vi "Graph_Peak_testing.vi"(0 "Channel Select":u16(ring) items=["Temperature"=9, "Flow/Min"=6, "Pressure_Bar"=3], 1 "CHL":T1={"chl1 MIN"=110.0, "chl1 MAX"=130.0, "chl1 thrshold"=120.0}, 5 "error in":errorcluster, 6 "CSV file path":path) -> (7 "samples count":i32, 9 "Max or peak value":ext[](array[numeric]), 10 "size(s)":i32, 11 "Min or Valley value":ext[](array[numeric]), 12 "Peak_valley_point":ext[](array[numeric]), 13 "Peak_valley_point_time":timestamp[](array[timestamp]), 14 "Max Valley/Min":dbl, 15 "XY Graph 2":cluster{timestamp[], ext[]}(graph), 17 "Min Valley/Min":dbl, 18 "Peak or Valley Fail":bool, 19 "error out":errorcluster)   [LabVIEW 2017]
uses:
  <vilib>/Utility/miscctls.llb/LVCursorListTypeDef.ctl
  <vilib>/Utility/file.llb/Read Delimited Spreadsheet (string).vi
  <userlib>/_OpenG.lib/array/array.llb/Remove Duplicates from 1D Array (Variant)__ogtk.vi
  <userlib>/_OpenG.lib/array/array.llb/Delete Elements from 1D Array (EXT)__ogtk.vi
panel:
  out "size(s) 5":i32
  out "array w/ subset deleted":ext[](array[numeric]) format="%.2f"
  out "indices of removed elements":i32[](array[numeric])
  out "size(s) 3":i32
  out "Numeric 3":i32
  out "Numeric":i32
  out "Array 13":ext[][](array[numeric])
  out "Array 12":ext[](array[numeric])
  out "deleted portion 2":ext[](array[numeric])
  out "appended array 2":timestamp[][](array[timestamp])
  out "size(s) 2":i32
  out "Array 11":ext[](array[numeric])
  out "Array 8":timestamp[](array[timestamp])
  out "appended array":timestamp[][](array[timestamp])
  out "deleted portion":ext[](array[numeric])
  out "Array 10":ext[](array[numeric])
  out "Array 9":ext[][](array[numeric])
  out "output cluster 3":T2(array[cluster])
  in  "Cursor List 3":T3
  out "Numeric 2":i32
  out "x = y?":bool
  out "x+y 2":i32
  out "STOP THRESHOLD TRIGGER":i32
  out "START THRESHOLD TRIGGER":i32
  out "time stamp":timestamp[](array[timestamp])
  out "number":ext[](array[numeric])
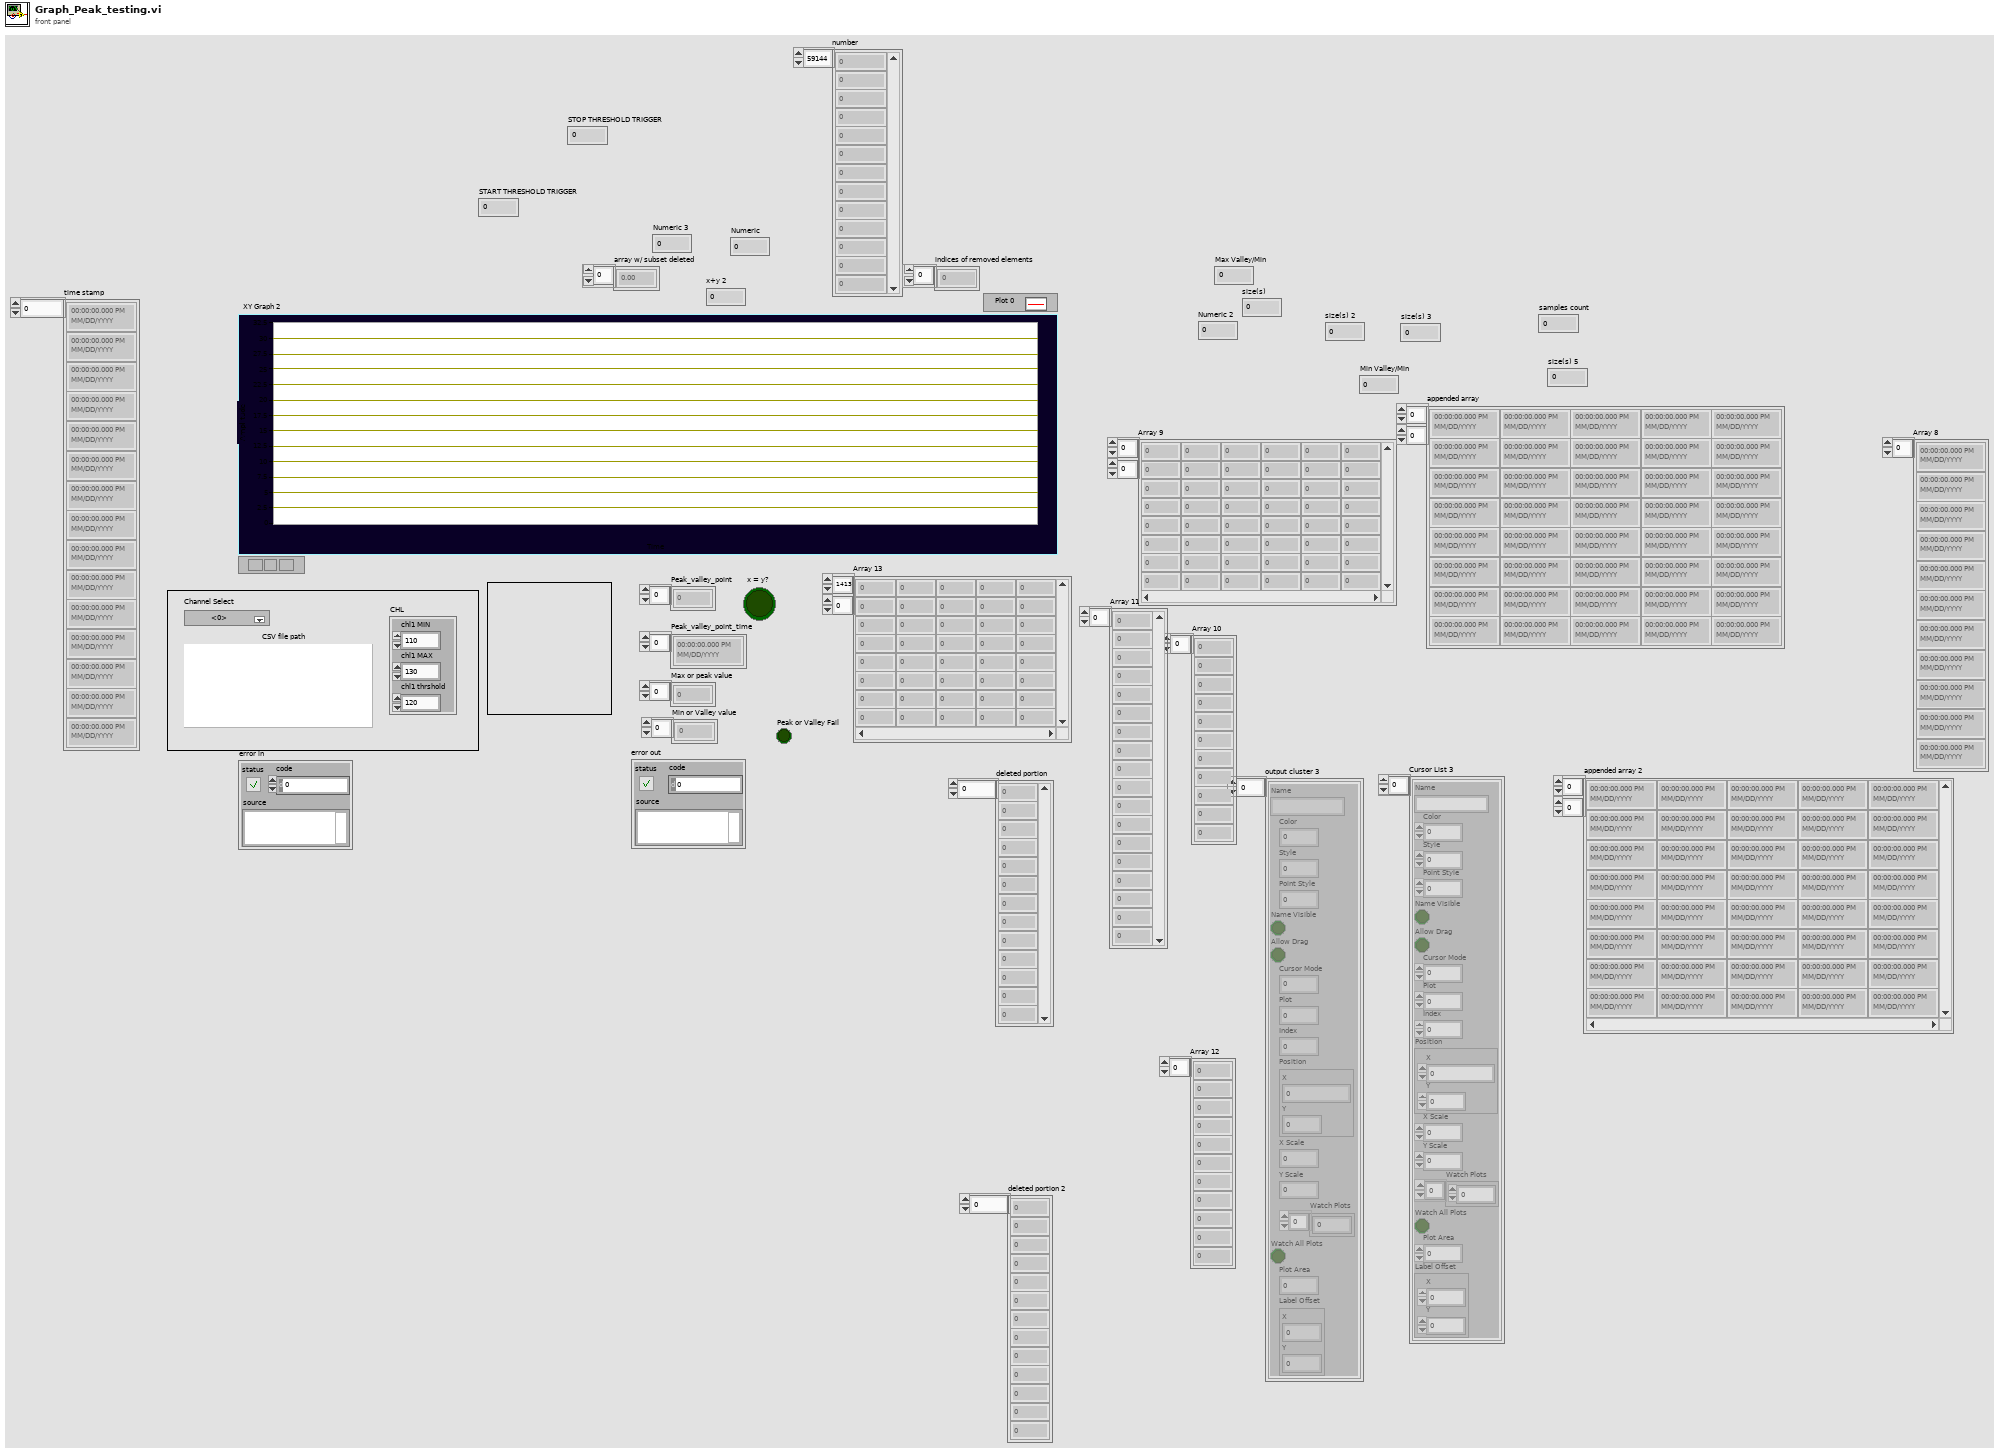
[diagram p1: front panel]
types:
  T1 = cluster{"chl1 MIN":dbl, "chl1 MAX":dbl, "chl1 thrshold":dbl}
  T2 = cluster{"Name":string, "Color":u32, "Style":u8, "Point Style":u8, "Name Visible":bool, "Allow Drag":bool, "Cursor Mode":u32, "Plot":i32, "Index":i32, "Position":cluster{"X":dbl, "Y":dbl}, "X Scale":u32, "Y Scale":u32, "Watch Plots":i32[], "Watch All Plots":bool, "Plot Area":i32, "Label Offset":cluster{"X":dbl, "Y":dbl}}[]
  T3 = typedef "LVCursorListTypeDef.ctl" = cluster{"Name":string, "Color":u32, "Style":u8, "Point Style":u8, "Name Visible":bool, "Allow Drag":bool, "Cursor Mode":u32, "Plot":i32, "Index":i32, "Position":cluster{"X":dbl, "Y":dbl}, "X Scale":u32, "Y Scale":u32, "Watch Plots":i32[], "Watch All Plots":bool, "Plot Area":i32, "Label Offset":cluster{"X":dbl, "Y":dbl}}[]
  T4 = typedef "LVDateTimeRec.ctl" = cluster{"fractional second":dbl, "second":i32, "minute":i32, "hour":i32, "day of month":i32, "month":i32, "year":i32, "day of week":i32, "day of year":i32, "DST":i32}
  T5 = cluster{"Name":string, "Color":u32, "Style":u8, "Point Style":u8, "Name Visible":bool, "Allow Drag":bool, "Cursor Mode":u32, "Plot":i32, "Index":i32, "Position":cluster{"X":dbl, "Y":dbl}, "X Scale":u32, "Y Scale":u32, "Watch Plots":i32[], "Watch All Plots":bool, "Plot Area":i32, "Label Offset":cluster{"X":dbl, "Y":dbl}}
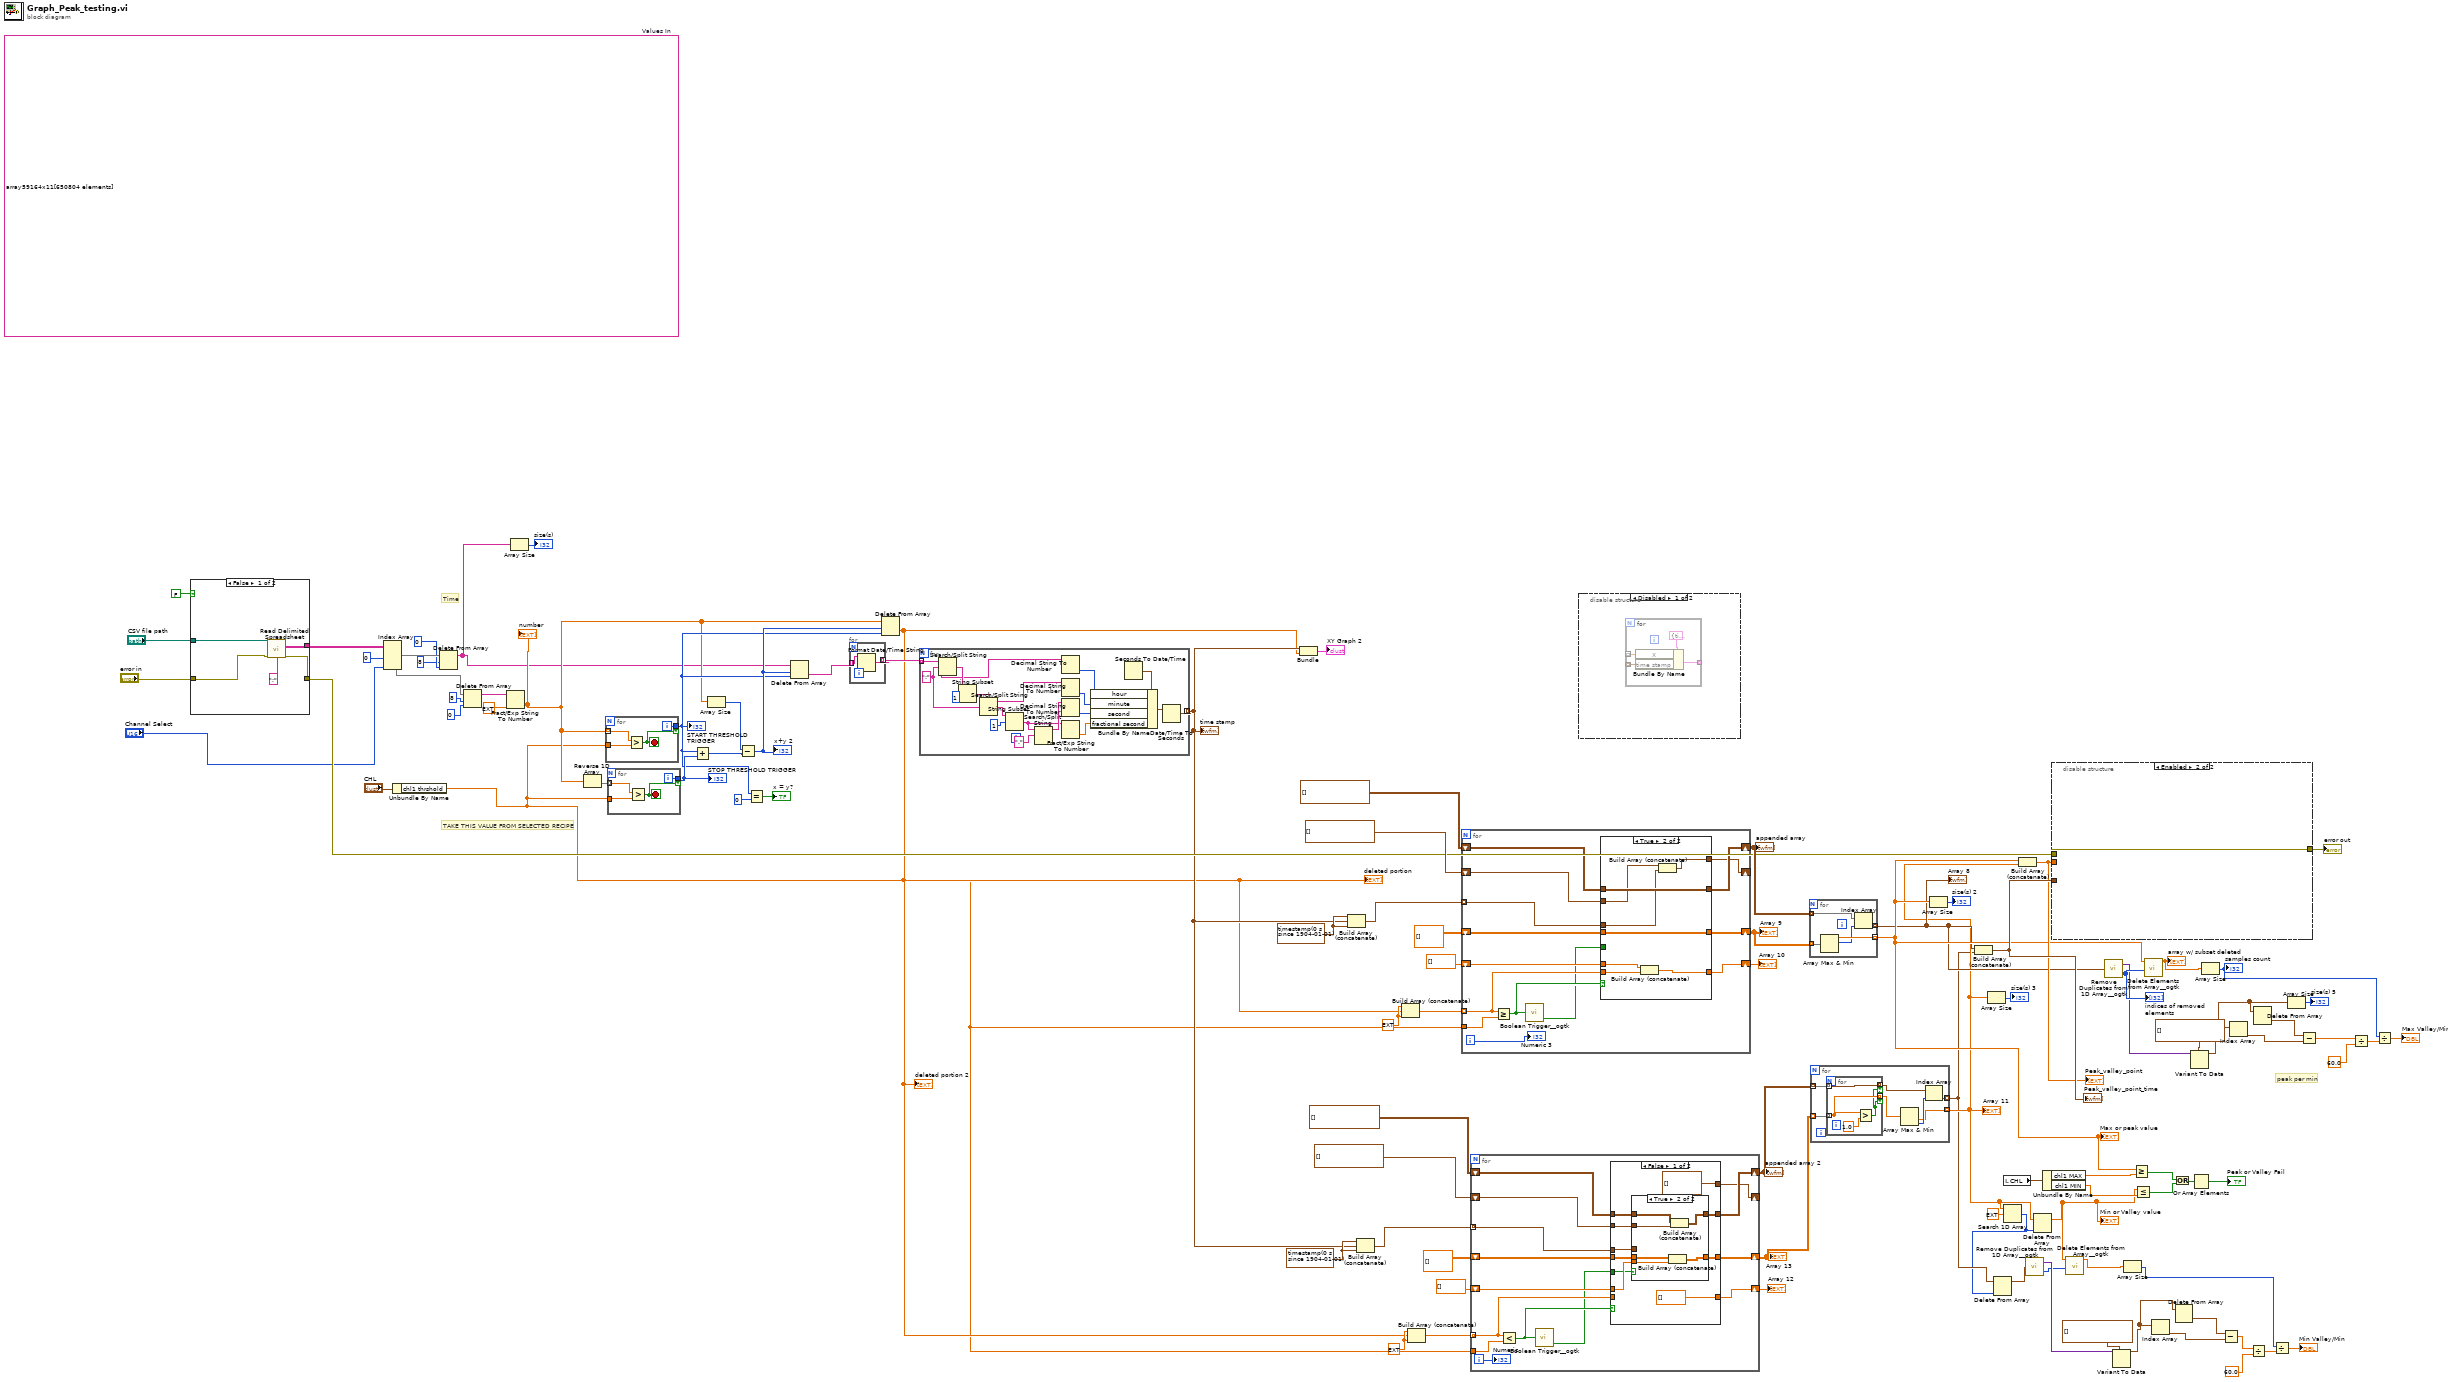
[diagram p0: block diagram]
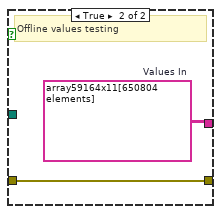
[diagram p3: hidden frame]
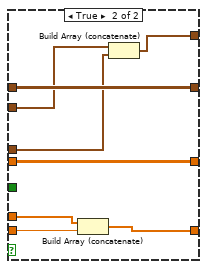
[diagram p5: hidden frame]
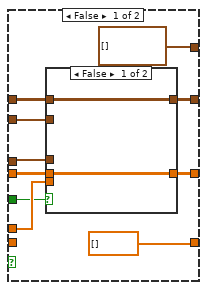
[diagram p6: hidden frame]
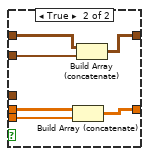
[diagram p7: hidden frame]
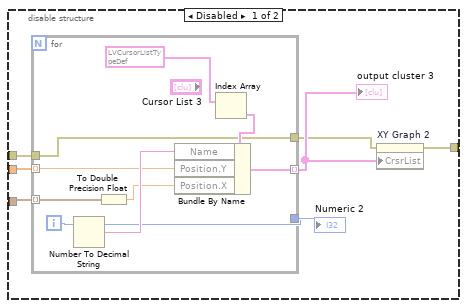
[diagram p8: hidden frame]
diagram:
  (unwired) string[][] array59164x11[650804 elements]  # Values In
  w66 = timestamp(0 s since 1904-01-01) ("time stamp")
  w65 = ext 0.0 ("String")
  w76 = timestamp(0 s since 1904-01-01) ("time stamp")
  w77 = ext 0.0 ("String")
  # "peak per min"
  # "Time"
  # "TAKE THIS VALUE FROM SELECTED RECIPE"
  n1 = case shown="False" FALSE {
    tunnel: [w104 w107] -> w95
    tunnel: "CSV file path" -> [w103 _]
    tunnel: [w102 w106] -> w53
    tunnel: "error in" -> [w101 w106]
    frame False {
      n2 = call-poly <vilib>:"Read Delimited Spreadsheet.vi"("file path (dialog if empty)"=w103, "error in (no error)"=w101, "delimiter (\\t)"=";" ("delimiter (\\t)")) -> ("all rows"=w104:string[][], "error out"=w102:errorcluster)  [unwired: 7 in, 4 out]
    }
    frame True {
      w107 = string[][] array59164x11[650804 elements]  # Values In
      # "Offline values testing"
    }
  }
  n3 = Index Array(array=w95, index (col) #1=0 ("index (row)"), index (col) #2="Channel Select") -> (element #1=w100:string[], element #2=w96:string[])  [unwired: 2 in]
  n4 = Unbundle By Name("CHL") -> ("chl1 thrshold"=w44:dbl)
  n5 = Delete From Array(array=w100, length=8 ("index (row)"), index=0 ("index (row)")) -> (array with subset deleted=w8:string[])  [unwired: 1 out]
  n6 = Delete From Array(array=w96, length=8 ("index (row)"), index=0 ("index (row)")) -> (array with subset deleted=w90:string[])  [unwired: 1 out]
  n7 = Fract/Exp String To Number(string=w90, default (0 dbl)=ext 0.0 ("String")) -> (number=w48:ext[])  [unwired: 2 in, 1 out]
  "number" <- w48
  n8 = Array Size(array=w8) -> (size(s)=→"size(s)":i32)
  n9 = Reverse 1D Array(array=w48) -> (reversed array=w89:ext[])
  n10 = for {
    tunnel: w48 -> [w111] mode=indexing
    tunnel: [w110] -> w84 if=w109
    tunnel: w44 -> [w108]
    i -> [w110]
    stop <- w109 stop-if-true
    n11 = Greater?(x=w111, y=w108) -> (0:w109:bool)
  }
  "START THRESHOLD TRIGGER" <- w84
  n12 = for {
    tunnel: w89 -> [w115] mode=indexing
    tunnel: [w114] -> w88 if=w113
    tunnel: w44 -> [w112]
    i -> [w114]
    stop <- w113 stop-if-true
    n13 = Greater?(x=w115, y=w112) -> (0:w113:bool)
  }
  "STOP THRESHOLD TRIGGER" <- w88
  n14 = Add(x=w84, y=w88) -> (x+y=w86:i32)
  n15 = Array Size(array=w48) -> (size(s)=w87:i32)
  n16 = Subtract(x=w87, y=w86) -> (x-y=w85:i32)
  "x+y 2" <- w85
  n17 = Equal?(x=w84, y=0) -> (x = y?=→"x = y?":bool)
  n18 = Delete From Array(array=w8, length=w85, index=w84) -> (deleted portion=w46:string[])  [unwired: 1 out]
  n19 = for {
    tunnel: w46 -> [w117] mode=indexing
    tunnel: [w116] -> w92 mode=indexing
    n20 = Format Date/Time String(time format string (%c)=w117) -> (date/time string=w116:string)  [unwired: 2 in]
  }
  n21 = Delete From Array(array=w48, length=w85, index=w84) -> (deleted portion=w47:ext[])  [unwired: 1 out]
  "deleted portion" <- w47
  "deleted portion 2" <- w47
  n22 = for {
    tunnel: w92 -> [w126] mode=indexing
    tunnel: [w134] -> w50 mode=indexing
    w133 = ":" ("format string")
    n23 = Search/Split String(string=w126, search string/char (-)=w133) -> (substring before match=w122:string, match + rest of string=w131:string)  [unwired: 1 in, 1 out]
    n24 = String Subset(string=w131, offset (0)=1) -> (substring=w130:string)  [unwired: 1 in]
    n25 = Search/Split String(string=w130, search string/char (-)=w133) -> (substring before match=w121:string, match + rest of string=w128:string)  [unwired: 1 in, 1 out]
    n26 = String Subset(string=w128, offset (0)=1) -> (substring=w120:string)  [unwired: 1 in]
    n27 = Search/Split String(string=w120, search string/char (-)="." ("format string")) -> (substring before match=w125:string)  [unwired: 1 in, 2 out]
    n28 = Decimal String To Number(string=w122) -> (number=w123:i32)  [unwired: 2 in, 1 out]
    n29 = Decimal String To Number(string=w121) -> (number=w124:i32)  [unwired: 2 in, 1 out]
    n30 = Decimal String To Number(string=w125) -> (number=w118:i32)  [unwired: 2 in, 1 out]
    n31 = Fract/Exp String To Number(string=w120) -> (number=w119:dbl)  [unwired: 3 in, 1 out]
    n32 = Seconds To Date/Time() -> (date time rec=w135:T4)  [unwired: 2 in]
    n33 = Bundle By Name(cluster=w135, "hour"=w123, "minute"=w124, "second"=w118, "fractional second"=w119) -> (w136:T4)
    n34 = Date/Time To Seconds(2:w136) -> (0:w134:timestamp)  [unwired: 1 in]
  }
  "time stamp" <- w50
  n35 = Bundle(w50, w47) -> (→"XY Graph 2":cluster{timestamp[], ext[]})  [unwired: 1 in]
  n36 = Build Array (concatenate)(w76, w50, w76) -> (w73:timestamp[])
  n37 = Build Array (concatenate)(w66, w50, w66) -> (w69:timestamp[])
  n38 = Build Array (concatenate)(w77, w47, w77) -> (w78:ext[])
  n39 = Build Array (concatenate)(w65, w47, w65) -> (w64:ext[])
  n40 = for {
    tunnel: w78 -> [w148] mode=indexing
    tunnel: w44 -> [w150]
    shift-right: [w147] -> w79
    shift-left: ext[] [] -> [w146]
    shift-right: [w144] -> w72
    shift-left: ext[][] [] -> [w145]
    tunnel: w73 -> [w142] mode=indexing
    shift-right: [w141] -> w71
    shift-left: timestamp[][] [] ("appended array") -> [w140]
    shift-right: [w138] -> _
    shift-left: timestamp[] [] ("appended array") -> [w139]
    i -> [w137]
    n41 = Greater Or Equal?(x=w148, y=w150) -> (x >= y?=w149:bool)
    n42 = call <userlib>:"Boolean Trigger__ogtk.vi"("Boolean Input"=w149) -> ("Falling Edge"=w143:bool)  [unwired: 1 in, 1 out]
    n43 = case shown="True" w149 {
      tunnel: w148 -> [_ w176]
      tunnel: [ext[] [] w175] -> w147
      tunnel: w146 -> [w157 w173]
      tunnel: w145 -> [w158 w174]
      tunnel: [w159 w174] -> w144
      tunnel: w143 -> [w156 _]
      tunnel: w142 -> [w155 w169]
      tunnel: [w154 w172] -> w141
      tunnel: w140 -> [w153 w172]
      tunnel: w139 -> [w152 w170]
      tunnel: [timestamp[] [] ("appended array") w171] -> w138
      frame False {
        n44 = case shown="False" w156 {
          tunnel: [w162 w168] -> w159
          tunnel: w158 -> [w162 w167]
          tunnel: w157 -> [_ w166]
          tunnel: w155 -> [_ _]
          tunnel: [w161 w165] -> w154
          tunnel: w153 -> [w161 w164]
          tunnel: w152 -> [_ w163]
          frame False {
          }
          frame True {
            n45 = Build Array (concatenate)(w167, w166) -> (w168:ext[][])
            n46 = Build Array (concatenate)(w164, w163) -> (w165:timestamp[][])
          }
        }
      }
      frame True {
        n47 = Build Array (concatenate)(w173, w176) -> (w175:ext[])
        n48 = Build Array (concatenate)(w170, w169) -> (w171:timestamp[])
      }
    }
    "Numeric 3" <- w137
  }
  "Array 9" <- w72
  "Array 10" <- w79
  "appended array" <- w71
  n49 = for {
    tunnel: w64 -> [w188] mode=indexing
    tunnel: w44 -> [w190]
    shift-right: [w187] -> w63
    shift-left: ext[] [] -> [w186]
    shift-right: [w184] -> w58
    shift-left: ext[][] [] -> [w185]
    tunnel: w69 -> [w182] mode=indexing
    shift-right: [w181] -> w57
    shift-left: timestamp[][] [] ("appended array") -> [w180]
    shift-right: [w178] -> _
    shift-left: timestamp[] [] ("appended array") -> [w179]
    i -> [w177]
    n50 = Less?(x=w188, y=w190) -> (x < y?=w189:bool)
    n51 = call <userlib>:"Boolean Trigger__ogtk.vi"("Boolean Input"=w189) -> ("Falling Edge"=w183:bool)  [unwired: 1 in, 1 out]
    n52 = case shown="False" w189 {
      tunnel: w188 -> [_ w216]
      tunnel: [ext[] [] w215] -> w187
      tunnel: w186 -> [w197 w213]
      tunnel: w185 -> [w198 w214]
      tunnel: [w199 w214] -> w184
      tunnel: w183 -> [w196 _]
      tunnel: w182 -> [w195 w209]
      tunnel: [w194 w212] -> w181
      tunnel: w180 -> [w193 w212]
      tunnel: w179 -> [w192 w210]
      tunnel: [timestamp[] [] ("appended array") w211] -> w178
      frame False {
        n53 = case shown="True" w196 {
          tunnel: [w202 w208] -> w199
          tunnel: w198 -> [w202 w207]
          tunnel: w197 -> [_ w206]
          tunnel: w195 -> [_ _]
          tunnel: [w201 w205] -> w194
          tunnel: w193 -> [w201 w204]
          tunnel: w192 -> [_ w203]
          frame False {
          }
          frame True {
            n54 = Build Array (concatenate)(w207, w206) -> (w208:ext[][])
            n55 = Build Array (concatenate)(w204, w203) -> (w205:timestamp[][])
          }
        }
      }
      frame True {
        n56 = Build Array (concatenate)(w213, w216) -> (w215:ext[])
        n57 = Build Array (concatenate)(w210, w209) -> (w211:timestamp[])
      }
    }
    "Numeric" <- w177
  }
  "Array 13" <- w58
  "Array 12" <- w63
  "appended array 2" <- w57
  n58 = disable-structure shown="Disabled" {
    frame Disabled {
      n59 = for {
        tunnel: _ -> [w217] mode=indexing
        tunnel: [w220] -> _ mode=indexing
        tunnel: _ -> [w218] mode=indexing
        n60 = Bundle By Name(cluster=cluster{"time stamp":timestamp, "X":dbl} {"time stamp"=timestamp(0 s since 1904-01-01), "X"=0.0}, "X"=w217, "time stamp"=w218) -> (w220:cluster{"time stamp":timestamp, "X":dbl})
      }
    }
    frame Enabled {
    }
  }
  n61 = for {
    tunnel: w72 -> [w225] mode=indexing
    tunnel: w71 -> [w223] mode=indexing
    tunnel: [w224] -> w34 mode=indexing
    tunnel: [w221] -> w24 mode=indexing
    n62 = Array Max & Min(array=w225) -> (max value=w224:ext, max index (indices)=w222:i32)  [unwired: 2 out]
    n63 = Index Array(array=w223, index=w222) -> (element=w221:timestamp)
  }
  "Array 8" <- w24
  "Max or peak value" <- w34
  n64 = for {
    tunnel: w58 -> [w227] mode=indexing
    tunnel: w57 -> [w229] mode=indexing
    tunnel: [w230] -> w5 mode=indexing
    tunnel: [w232] -> w3 mode=indexing
    n65 = for {
      tunnel: w227 -> [w234] mode=indexing
      tunnel: [w235] -> w228 mode=indexing if=w233
      tunnel: w229 -> [w235] mode=indexing
      tunnel: [w234] -> w226 mode=indexing if=w233
      n66 = Greater?(x=w234, y=1.0) -> (0:w233:bool)
    }
    n67 = Array Max & Min(array=w226) -> (min value=w230:ext, min index (indices)=w231:i32)  [unwired: 2 out]
    n68 = Index Array(array=w228, index=w231) -> (element=w232:timestamp)
  }
  "Array 11" <- w5
  n69 = Array Size(array=w34) -> (size(s)=→"size(s) 2":i32)
  n70 = Build Array (concatenate)(w24, w3) -> (w60:timestamp[])
  "Peak_valley_point_time" <- w60
  n71 = Array Size(array=w5) -> (size(s)=→"size(s) 3":i32)
  n72 = local read "CHL"() -> (w42:T1)
  n73 = Search 1D Array(1D array=w5, element=ext 0.0) -> (index of element=w2:i32)  [unwired: 1 in]
  n74 = Delete From Array(array=w3, index=w2) -> (array with subset deleted=w1:timestamp[])  [unwired: 1 in, 1 out]
  n75 = Build Array (concatenate)(w34, w5) -> (w59:ext[])
  "Peak_valley_point" <- w59
  n76 = call-poly <userlib>:"Remove Duplicates from 1D Array__ogtk.vi"("Input Array"=w1) -> ("Output Array"=w13:variant[], "indices of removed elements"=w10:i32[])
  n77 = Delete From Array(array=w5, index=w2) -> (array with subset deleted=w4:ext[])  [unwired: 1 in, 1 out]
  "Min or Valley value" <- w4
  n78 = Unbundle By Name(w42) -> ("chl1 MAX"=w41:dbl, "chl1 MIN"=w40:dbl)
  n79 = disable-structure shown="Enabled" {
    disable-tunnel: w59 -> [w241 _]
    disable-tunnel: w60 -> [w240 _]
    disable-tunnel: w53 -> [w238 w253]
    disable-tunnel: [w237 w253] -> w51
    frame Disabled {
      n80 = for {
        tunnel: [w251] -> w242 mode=indexing
        tunnel: [w248] -> w243
        tunnel: w240 -> [w246] mode=indexing
        tunnel: w241 -> [w245] mode=indexing
        tunnel: [w244] -> w239
        tunnel: w238 -> [w244]
        i -> [w248]
        n81 = Number To Decimal String(number=w248) -> (decimal integer string=w250:string)  [unwired: 1 in]
        n82 = To Double Precision Float(number=w246) -> (double precision float=w249:dbl)
        n83 = Index Array(array=T3 [{"Name"="0", "Color"=0, "Style"=0, "Point Style"=13, "Name Visible"=FALSE, "Allow Drag"=FALSE, "Cursor Mode"=0, "Plot"=0, "Index"=0, "Position"={"X"=3725289003.72, "Y"=121.765}, "X Scale"=0, "Y Scale"=0, "Watch Plots"=[], "Watch All Plots"=FALSE, "Plot Area"=0, "Label Offset"={"X"=0.0, "Y"=0.0}}, {"Name"="1", "Color"=0, "Style"=0, "Point Style"=0, "Name Visible"=FALSE, "Allow Drag"=FALSE, "Cursor Mode"=0, "Plot"=0, "Index"=0, "Position"={"X"=3725289003.725, "Y"=125.02090909090909}, "X Scale"=0, "Y Scale"=0, "Watch Plots"=[], "Watch All Plots"=FALSE, "Plot Area"=0, "Label Offset"={"X"=0.0, "Y"=0.0}}, {"Name"="2", "Color"=0, "Style"=0, "Point Style"=0, "Name Visible"=FALSE, "Allow Drag"=FALSE, "Cursor Mode"=0, "Plot"=0, "Index"=0, "Position"={"X"=3725289003.728, "Y"=128.01}, "X Scale"=0, "Y Scale"=0, "Watch Plots"=[], "Watch All Plots"=FALSE, "Plot Area"=0, "Label Offset"={"X"=0.0, "Y"=0.0}}, {"Name"="3", "Color"=0, "Style"=0, "Point Style"=0, "Name Visible"=FALSE, "Allow Drag"=FALSE, "Cursor Mode"=0, "Plot"=0, "Index"=0, "Position"={"X"=3725289003.73, "Y"=123.4901219512195}, "X Scale"=0, "Y Scale"=0, "Watch Plots"=[], "Watch All Plots"=FALSE, "Plot Area"=0, "Label Offset"={"X"=0.0, "Y"=0.0}}, {"Name"="4", "Color"=0, "Style"=0, "Point Style"=0, "Name Visible"=FALSE, "Allow Drag"=FALSE, "Cursor Mode"=0, "Plot"=0, "Index"=0, "Position"={"X"=3725289003.732, "Y"=120.435}, "X Scale"=0, "Y Scale"=0, "Watch Plots"=[], "Watch All Plots"=FALSE, "Plot Area"=0, "Label Offset"={"X"=0.0, "Y"=0.0}}, {"Name"="5", "Color"=0, "Style"=0, "Point Style"=0, "Name Visible"=FALSE, "Allow Drag"=FALSE, "Cursor Mode"=0, "Plot"=0, "Index"=0, "Position"={"X"=3725289003.752, "Y"=121.25480392156864}, "X Scale"=0, "Y Scale"=0, "Watch Plots"=[], "Watch All Plots"=FALSE, "Plot Area"=0, "Label Offset"={"X"=0.0, "Y"=0.0}}, {"Name"="6", "Color"=0, "Style"=0, "Point Style"=0, "Name Visible"=FALSE, "Allow Drag"=FALSE, "Cursor Mode"=0, "Plot"=0, "Index"=0, "Position"={"X"=3725289003.756, "Y"=123.92999999999999}, "X Scale"=0, "Y Scale"=0, "Watch Plots"=[], "Watch All Plots"=FALSE, "Plot Area"=0, "Label Offset"={"X"=0.0, "Y"=0.0}}, {"Name"="7", "Color"=0, "Style"=0, "Point Style"=0, "Name Visible"=FALSE, "Allow Drag"=FALSE, "Cursor Mode"=0, "Plot"=0, "Index"=0, "Position"={"X"=3725289003.762, "Y"=127.01970588235294}, "X Scale"=0, "Y Scale"=0, "Watch Plots"=[], "Watch All Plots"=FALSE, "Plot Area"=0, "Label Offset"={"X"=0.0, "Y"=0.0}}, {"Name"="8", "Color"=0, "Style"=0, "Point Style"=0, "Name Visible"=FALSE, "Allow Drag"=FALSE, "Cursor Mode"=0, "Plot"=0, "Index"=0, "Position"={"X"=3725289003.765, "Y"=131.29425531914893}, "X Scale"=0, "Y Scale"=0, "Watch Plots"=[], "Watch All Plots"=FALSE, "Plot Area"=0, "Label Offset"={"X"=0.0, "Y"=0.0}}, {"Name"="9", "Color"=0, "Style"=0, "Point Style"=0, "Name Visible"=FALSE, "Allow Drag"=FALSE, "Cursor Mode"=0, "Plot"=0, "Index"=0, "Position"={"X"=3725289003.767, "Y"=128.4116891891892}, "X Scale"=0, "Y Scale"=0, "Watch Plots"=[], "Watch All Plots"=FALSE, "Plot Area"=0, "Label Offset"={"X"=0.0, "Y"=0.0}}, {"Name"="10", "Color"=0, "Style"=0, "Point Style"=0, "Name Visible"=FALSE, "Allow Drag"=FALSE, "Cursor Mode"=0, "Plot"=0, "Index"=0, "Position"={"X"=3725289003.768, "Y"=122.84}, "X Scale"=0, "Y Scale"=0, "Watch Plots"=[], "Watch All Plots"=FALSE, "Plot Area"=0, "Label Offset"={"X"=0.0, "Y"=0.0}}, {"Name"="11", "Color"=0, "Style"=0, "Point Style"=0, "Name Visible"=FALSE, "Allow Drag"=FALSE, "Cursor Mode"=0, "Plot"=0, "Index"=0, "Position"={"X"=3725289003.794, "Y"=121.99}, "X Scale"=0, "Y Scale"=0, "Watch Plots"=[], "Watch All Plots"=FALSE, "Plot Area"=0, "Label Offset"={"X"=0.0, "Y"=0.0}}, {"Name"="12", "Color"=0, "Style"=0, "Point Style"=0, "Name Visible"=FALSE, "Allow Drag"=FALSE, "Cursor Mode"=0, "Plot"=0, "Index"=0, "Position"={"X"=3725289003.803, "Y"=128.6199504950495}, "X Scale"=0, "Y Scale"=0, "Watch Plots"=[], "Watch All Plots"=FALSE, "Plot Area"=0, "Label Offset"={"X"=0.0, "Y"=0.0}}, {"Name"="13", "Color"=0, "Style"=0, "Point Style"=0, "Name Visible"=FALSE, "Allow Drag"=FALSE, "Cursor Mode"=0, "Plot"=0, "Index"=0, "Position"={"X"=3725289003.806, "Y"=132.86499999999998}, "X Scale"=0, "Y Scale"=0, "Watch Plots"=[], "Watch All Plots"=FALSE, "Plot Area"=0, "Label Offset"={"X"=0.0, "Y"=0.0}}, {"Name"="14", "Color"=0, "Style"=0, "Point Style"=0, "Name Visible"=FALSE, "Allow Drag"=FALSE, "Cursor Mode"=0, "Plot"=0, "Index"=0, "Position"={"X"=3725289003.808, "Y"=128.93437743190663}, "X Scale"=0, "Y Scale"=0, "Watch Plots"=[], "Watch All Plots"=FALSE, "Plot Area"=0, "Label Offset"={"X"=0.0, "Y"=0.0}}, {"Name"="15", "Color"=0, "Style"=0, "Point Style"=0, "Name Visible"=FALSE, "Allow Drag"=FALSE, "Cursor Mode"=0, "Plot"=0, "Index"=0, "Position"={"X"=3725289003.83, "Y"=121.8}, "X Scale"=0, "Y Scale"=0, "Watch Plots"=[], "Watch All Plots"=FALSE, "Plot Area"=0, "Label Offset"={"X"=0.0, "Y"=0.0}}, {"Name"="16", "Color"=0, "Style"=0, "Point Style"=0, "Name Visible"=FALSE, "Allow Drag"=FALSE, "Cursor Mode"=0, "Plot"=0, "Index"=0, "Position"={"X"=3725289003.84, "Y"=128.54500000000002}, "X Scale"=0, "Y Scale"=0, "Watch Plots"=[], "Watch All Plots"=FALSE, "Plot Area"=0, "Label Offset"={"X"=0.0, "Y"=0.0}}, {"Name"="17", "Color"=0, "Style"=0, "Point Style"=0, "Name Visible"=FALSE, "Allow Drag"=FALSE, "Cursor Mode"=0, "Plot"=0, "Index"=0, "Position"={"X"=3725289003.842, "Y"=129.14884615384614}, "X Scale"=0, "Y Scale"=0, "Watch Plots"=[], "Watch All Plots"=FALSE, "Plot Area"=0, "Label Offset"={"X"=0.0, "Y"=0.0}}, {"Name"="18", "Color"=0, "Style"=0, "Point Style"=0, "Name Visible"=FALSE, "Allow Drag"=FALSE, "Cursor Mode"=0, "Plot"=0, "Index"=0, "Position"={"X"=3725289003.845, "Y"=133.010296912114}, "X Scale"=0, "Y Scale"=0, "Watch Plots"=[], "Watch All Plots"=FALSE, "Plot Area"=0, "Label Offset"={"X"=0.0, "Y"=0.0}}, {"Name"="19", "Color"=0, "Style"=0, "Point Style"=0, "Name Visible"=FALSE, "Allow Drag"=FALSE, "Cursor Mode"=0, "Plot"=0, "Index"=0, "Position"={"X"=3725289003.847, "Y"=128.22329145728645}, "X Scale"=0, "Y Scale"=0, "Watch Plots"=[], "Watch All Plots"=FALSE, "Plot Area"=0, "Label Offset"={"X"=0.0, "Y"=0.0}}] ("Cursor List")) -> (element=w252:T5)  [unwired: 1 in]
        n84 = Bundle By Name(cluster=w252, "Name"=w250, "Position.Y"=w245, "Position.X"=w249) -> (w251:T5)
      }
      "output cluster 3" <- w242
      "Numeric 2" <- w243
      n85 = property on="XY Graph 2" class="XYGraph (strict)"(error in=w239, "CrsrList"=w242) -> (error out=w237:errorcluster)  [unwired: 1 in, 1 out]
    }
    frame Enabled {
    }
  }
  "error out" <- w51
  n86 = call-poly <userlib>:"Delete Elements from Array__ogtk.vi"("indices"=w10, "array"=w4) -> ("array w/ subset deleted"=w11:ext[])  [unwired: 8 in, 1 out]
  n87 = call-poly <userlib>:"Remove Duplicates from 1D Array__ogtk.vi"("Input Array"=w24) -> ("Output Array"=w30:variant[], "indices of removed elements"=w35:i32[])
  "indices of removed elements" <- w35
  n88 = Variant To Data(type=timestamp[] [], Variant=w13) -> (data=w14:timestamp[])  [unwired: 1 in, 1 out]
  n89 = Array Size(array=w11) -> (size(s)=w18:i32)
  n90 = Greater Or Equal?(x=w34, y=w41) -> (x >= y?=w39:bool[])
  n91 = Less Or Equal?(x=w4, y=w40) -> (x <= y?=w38:bool[])
  n92 = call-poly <userlib>:"Delete Elements from Array__ogtk.vi"("indices"=w35, "array"=w34) -> ("array w/ subset deleted"=w33:ext[])  [unwired: 8 in, 1 out]
  "array w/ subset deleted" <- w33
  n93 = Index Array(array=w14) -> (element=w15:timestamp)  [unwired: 1 in]
  n94 = Or(x=w39, y=w38) -> (x .or. y?=w37:bool[])
  n95 = Delete From Array(array=w14) -> (deleted portion=w16:timestamp)  [unwired: 2 in, 1 out]
  n96 = Variant To Data(type=timestamp[] [], Variant=w30) -> (data=w29:timestamp[])  [unwired: 1 in, 1 out]
  n97 = Or Array Elements(Boolean array=w37) -> (logical OR=→"Peak or Valley Fail":bool)
  n98 = Array Size(array=w33) -> (size(s)=w23:i32)
  "samples count" <- w23
  n99 = Subtract(x=w16, y=w15) -> (x-y=w17:dbl)
  n100 = Index Array(array=w29) -> (element=w28:timestamp)  [unwired: 1 in]
  n101 = Divide(x=w17, y=60.0) -> (x/y=w19:dbl)
  n102 = Delete From Array(array=w29) -> (deleted portion=w27:timestamp)  [unwired: 2 in, 1 out]
  n103 = Divide(x=w18, y=w19) -> (x/y=→"Min Valley/Min":dbl)
  n104 = Array Size(array=w29) -> (size(s)=→"size(s) 5":i32)
  n105 = Subtract(x=w27, y=w28) -> (x-y=w26:dbl)
  n106 = Divide(x=w26, y=60.0) -> (x/y=w22:dbl)
  n107 = Divide(x=w23, y=w22) -> (x/y=→"Max Valley/Min":dbl)
